vi "GetCorrdinateSysForImageArray.vi"(0 "Result data in":T2={"Measurement Names Array"=[], "Pass-Fail Array"=[], "Measurement Values Array "=[], "Roi for overlay (Arrows) Array"=[], "Algo Type Array"=[], "Image Array"=[], "Clamp operations"=enum."Average Clamp", "  Search Direction "=[], "Images_Array_in"=[], "ResultPF"=FALSE, "Total Cluster Values"={"Total Fail"=0, "Total Pass"=0, "Total Count"=0}, "Reel Counter Cluster"={"Reel Fail"=0, "Reel Pass"=0, "Reel Count"=0}, "Tolerance  Array"=[], "Array of Cam Spec Control Bool"=[], "Control Pass Fail Array"=[], "Specification Pass Fail Array"=[], "Overlay Arrow Lines"=[], "Camera ID"=[], "Trigger count"=0, "Specification fail?"=FALSE}, 2 "ImageStreams":T4, 6 "error in":errorcluster) -> (21 "Co ordinate Other":T1, 22 "Co-Ordinate System":T5(array[cluster]), 25 "Result data out":T2={"Measurement Names Array"=[], "Pass-Fail Array"=[], "Measurement Values Array "=[], "Roi for overlay (Arrows) Array"=[], "Algo Type Array"=[], "Image Array"=[], "Clamp operations"=enum."Average Clamp", "  Search Direction "=[], "Images_Array_in"=[], "ResultPF"=FALSE, "Total Cluster Values"={"Total Fail"=0, "Total Pass"=0, "Total Count"=0}, "Reel Counter Cluster"={"Reel Fail"=0, "Reel Pass"=0, "Reel Count"=0}, "Tolerance  Array"=[], "Array of Cam Spec Control Bool"=[], "Control Pass Fail Array"=[], "Specification Pass Fail Array"=[], "Overlay Arrow Lines"=[], "Camera ID"=[], "Trigger count"=0, "Specification fail?"=FALSE}, 26 "error out":errorcluster)   [LabVIEW 2019, in "Algorithm.lvclass"]
uses:
  FrameworkOverrides/Algorithm.lvclass
  <vilib>/vision/Measure.llb/Edge Polarity.ctl
  <vilib>/vision/Measure.llb/Edge Options.ctl
  Controls/Result Cluster.ctl
  Controls/ImageStreams Type Def.ctl
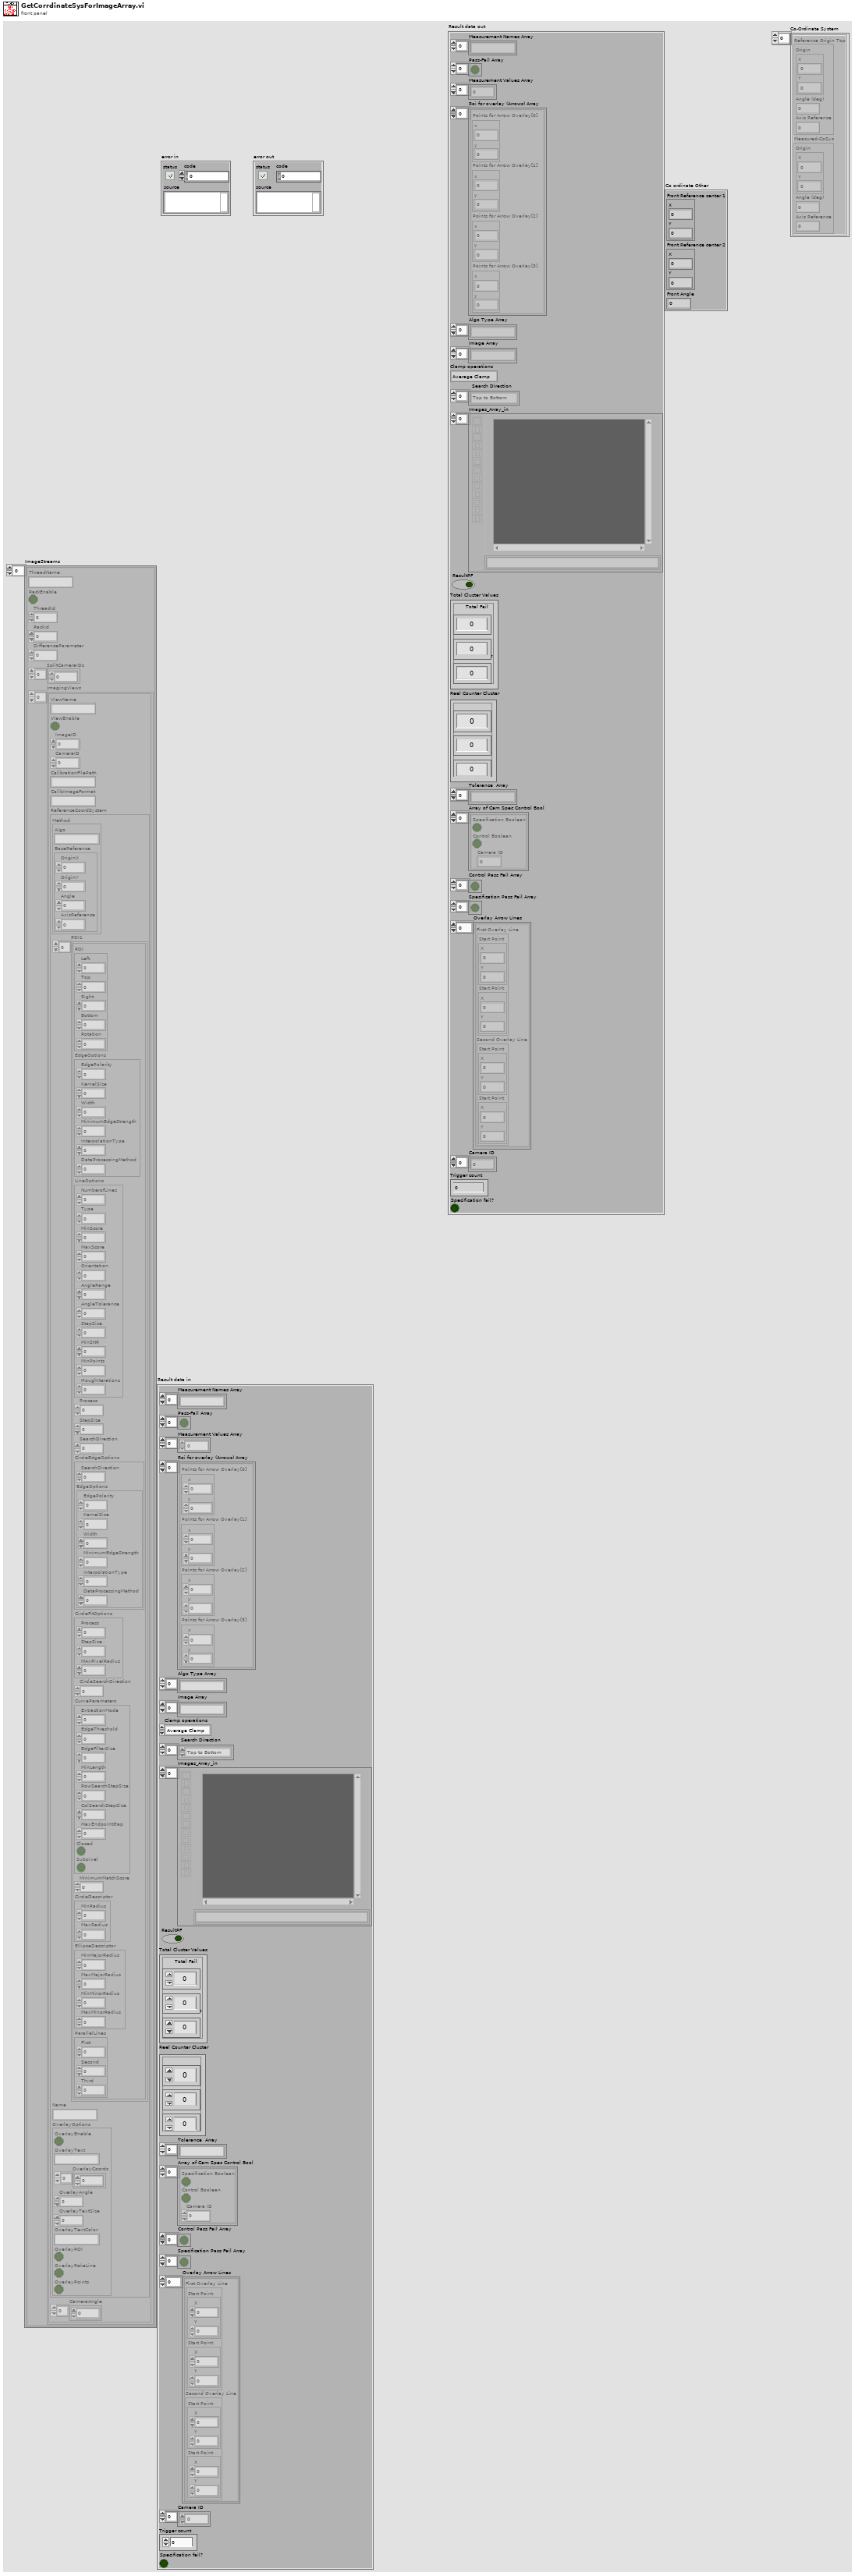
[diagram p1: front panel]
types:
  T1 = cluster{"Front Reference center 1":cluster{"X":sgl, "Y":sgl}, "Front Reference center 2":cluster{"X":sgl, "Y":sgl}, "Front Angle":dbl}
  T2 = typedef "Algorithm.lvclass/Result Cluster.ctl" = cluster{"Measurement Names Array":string[], "Pass-Fail Array":bool[], "Measurement Values Array ":dbl[], "Roi for overlay (Arrows) Array":cluster{"Points for Arrow Overlay[0]":cluster{"x":dbl, "y":dbl}, "Points for Arrow Overlay[1]":cluster{"x":dbl, "y":dbl}, "Points for Arrow Overlay[2]":cluster{"x":dbl, "y":dbl}, "Points for Arrow Overlay[3]":cluster{"x":dbl, "y":dbl}}[], "Algo Type Array":string[], "Image Array":string[], "Clamp operations":enum16{"Min Clamp", "Max Clamp", "Average Clamp"}, "  Search Direction ":enum16{"Left to Right", "Right to Left", "Top to Bottom", "Bottom to Top"}[], "Images_Array_in":T3[], "ResultPF":bool, "Total Cluster Values":cluster{"Total Fail":u64, "Total Pass":u64, "Total Count":u64}, "Reel Counter Cluster":cluster{"Reel Fail":u64, "Reel Pass":u64, "Reel Count":u64}, "Tolerance  Array":string[], "Array of Cam Spec Control Bool":cluster{"Specification Boolean":bool, "Control Boolean":bool, "Camera ID":i8}[], "Control Pass Fail Array":bool[], "Specification Pass Fail Array":bool[], "Overlay Arrow Lines":cluster{"First Overlay Line ":cluster{"Start Point":cluster{"X":sgl, "Y":sgl}, "Start Point":cluster{"X":sgl, "Y":sgl}}, "Second Overlay Line ":cluster{"Start Point":cluster{"X":sgl, "Y":sgl}, "Start Point":cluster{"X":sgl, "Y":sgl}}}[], "Camera ID":i8[], "Trigger count":i32, "Specification fail?":bool}
  T3 = typedef "IMAQ Image.ctl" = refnum<image>
  T4 = typedef "Algorithm.lvclass/ImageStreams Type Def.ctl" = cluster{"ThreadName":string, "RackEnable":bool, "ThreadId":i32, "RackId":i32, "DifferenceParameter":i32, "SplitCameraIDs":i32[], "ImagingViews":cluster{"ViewName":string, "ViewEnable":bool, "ImageID":i32, "CameraID":i32, "CalibrationFilePath":string, "CalibImageFormat":string, "ReferenceCoordSystem":cluster{"Method":cluster{"Algo":string, "BaseReference":cluster{"OriginX":i32, "OriginY":i32, "Angle":dbl, "AxisReference":i32}}, "ROI1":cluster{"ROI":cluster{"Left":i32, "Top":i32, "Right":i32, "Bottom":i32, "Rotation":dbl}, "EdgeOptions":cluster{"EdgePolarity":i32, "KernelSize":i32, "Width":i32, "MinimumEdgeStrength":i32, "InterpolationType":i32, "DataProcessingMethod":i32}, "LineOptions":cluster{"NumberofLines":i32, "Type":i32, "MinScore":i32, "MaxScore":i32, "Orientation":i32, "AngleRange":i32, "AngleTolerance":i32, "StepSize":i32, "MinSNR":i32, "MinPoints":i32, "HoughIterations":i32}, "Process":i32, "StepSize":i32, "SearchDirection":i32, "CircleEdgeOptions":cluster{"SearchDirection":i32, "EdgeOptions":cluster{"EdgePolarity":i32, "KernelSize":i32, "Width":i32, "MinimumEdgeStrength":i32, "InterpolationType":i32, "DataProcessingMethod":i32}}, "CircleFitOptions":cluster{"Process":i32, "StepSize":i32, "MAxPixelRadius":i32}, "CircleSearchDirection":i32, "CurveParameters":cluster{"ExtractionMode":i32, "EdgeThreshold":i32, "EdgeFilterSize":i32, "MinLength":i32, "RowSearchStepSize":i32, "ColSearchStepSize":i32, "MaxEndpointGap":i32, "Closed":bool, "Subpixel":bool}, "MinimumMatchScore":i32, "CircleDescriptor":cluster{"MinRadius":i32, "MaxRadius":i32}, "EllipseDescriptor":cluster{"MinMajorRadius":i32, "MaxMajorRadius":i32, "MinMinorRadius":i32, "MaxMinorRadius":i32}, "ParallelLines":cluster{"First":i32, "Second":i32, "Third":i32}}[], "Name":string, "OverlayOptions":cluster{"OverlayEnable":bool, "OverlayText":string, "OverlayCoords":i32[], "OverlayAngle":i32, "OverlayTextSize":i32, "OverlayTextColor":string, "OverlayROI":bool, "OverlayRakeLine":bool, "OverlayPoints":bool}}, "CameraAngle":dbl[]}[]}[]
  T5 = cluster{"Reference Origin Top":cluster{"Origin":cluster{"X":sgl, "Y":sgl}, "Angle (deg)":sgl, "Axis Reference":u32}, "Measured-CoSys":cluster{"Origin":cluster{"X":sgl, "Y":sgl}, "Angle (deg)":sgl, "Axis Reference":u32}}[]
  T6 = cluster{"ThreadName":string, "RackEnable":bool, "ThreadId":i32, "RackId":i32, "DifferenceParameter":i32, "SplitCameraIDs":i32[], "ImagingViews":cluster{"ViewName":string, "ViewEnable":bool, "ImageID":i32, "CameraID":i32, "CalibrationFilePath":string, "CalibImageFormat":string, "ReferenceCoordSystem":cluster{"Method":cluster{"Algo":string, "BaseReference":cluster{"OriginX":i32, "OriginY":i32, "Angle":dbl, "AxisReference":i32}}, "ROI1":cluster{"ROI":cluster{"Left":i32, "Top":i32, "Right":i32, "Bottom":i32, "Rotation":dbl}, "EdgeOptions":cluster{"EdgePolarity":i32, "KernelSize":i32, "Width":i32, "MinimumEdgeStrength":i32, "InterpolationType":i32, "DataProcessingMethod":i32}, "LineOptions":cluster{"NumberofLines":i32, "Type":i32, "MinScore":i32, "MaxScore":i32, "Orientation":i32, "AngleRange":i32, "AngleTolerance":i32, "StepSize":i32, "MinSNR":i32, "MinPoints":i32, "HoughIterations":i32}, "Process":i32, "StepSize":i32, "SearchDirection":i32, "CircleEdgeOptions":cluster{"SearchDirection":i32, "EdgeOptions":cluster{"EdgePolarity":i32, "KernelSize":i32, "Width":i32, "MinimumEdgeStrength":i32, "InterpolationType":i32, "DataProcessingMethod":i32}}, "CircleFitOptions":cluster{"Process":i32, "StepSize":i32, "MAxPixelRadius":i32}, "CircleSearchDirection":i32, "CurveParameters":cluster{"ExtractionMode":i32, "EdgeThreshold":i32, "EdgeFilterSize":i32, "MinLength":i32, "RowSearchStepSize":i32, "ColSearchStepSize":i32, "MaxEndpointGap":i32, "Closed":bool, "Subpixel":bool}, "MinimumMatchScore":i32, "CircleDescriptor":cluster{"MinRadius":i32, "MaxRadius":i32}, "EllipseDescriptor":cluster{"MinMajorRadius":i32, "MaxMajorRadius":i32, "MinMinorRadius":i32, "MaxMinorRadius":i32}, "ParallelLines":cluster{"First":i32, "Second":i32, "Third":i32}}[], "Name":string, "OverlayOptions":cluster{"OverlayEnable":bool, "OverlayText":string, "OverlayCoords":i32[], "OverlayAngle":i32, "OverlayTextSize":i32, "OverlayTextColor":string, "OverlayROI":bool, "OverlayRakeLine":bool, "OverlayPoints":bool}}, "CameraAngle":dbl[]}[]}
  T7 = cluster{"ViewName":string, "ViewEnable":bool, "ImageID":i32, "CameraID":i32, "CalibrationFilePath":string, "CalibImageFormat":string, "ReferenceCoordSystem":cluster{"Method":cluster{"Algo":string, "BaseReference":cluster{"OriginX":i32, "OriginY":i32, "Angle":dbl, "AxisReference":i32}}, "ROI1":cluster{"ROI":cluster{"Left":i32, "Top":i32, "Right":i32, "Bottom":i32, "Rotation":dbl}, "EdgeOptions":cluster{"EdgePolarity":i32, "KernelSize":i32, "Width":i32, "MinimumEdgeStrength":i32, "InterpolationType":i32, "DataProcessingMethod":i32}, "LineOptions":cluster{"NumberofLines":i32, "Type":i32, "MinScore":i32, "MaxScore":i32, "Orientation":i32, "AngleRange":i32, "AngleTolerance":i32, "StepSize":i32, "MinSNR":i32, "MinPoints":i32, "HoughIterations":i32}, "Process":i32, "StepSize":i32, "SearchDirection":i32, "CircleEdgeOptions":cluster{"SearchDirection":i32, "EdgeOptions":cluster{"EdgePolarity":i32, "KernelSize":i32, "Width":i32, "MinimumEdgeStrength":i32, "InterpolationType":i32, "DataProcessingMethod":i32}}, "CircleFitOptions":cluster{"Process":i32, "StepSize":i32, "MAxPixelRadius":i32}, "CircleSearchDirection":i32, "CurveParameters":cluster{"ExtractionMode":i32, "EdgeThreshold":i32, "EdgeFilterSize":i32, "MinLength":i32, "RowSearchStepSize":i32, "ColSearchStepSize":i32, "MaxEndpointGap":i32, "Closed":bool, "Subpixel":bool}, "MinimumMatchScore":i32, "CircleDescriptor":cluster{"MinRadius":i32, "MaxRadius":i32}, "EllipseDescriptor":cluster{"MinMajorRadius":i32, "MaxMajorRadius":i32, "MinMinorRadius":i32, "MaxMinorRadius":i32}, "ParallelLines":cluster{"First":i32, "Second":i32, "Third":i32}}[], "Name":string, "OverlayOptions":cluster{"OverlayEnable":bool, "OverlayText":string, "OverlayCoords":i32[], "OverlayAngle":i32, "OverlayTextSize":i32, "OverlayTextColor":string, "OverlayROI":bool, "OverlayRakeLine":bool, "OverlayPoints":bool}}, "CameraAngle":dbl[]}[]
  T8 = cluster{"Origin":cluster{"X":sgl, "Y":sgl}, "Angle (deg)":sgl, "Axis Reference":u32}
  T9 = cluster{"Base Reference":cluster{"Origin":cluster{"X":sgl, "Y":sgl}, "Angle (deg)":sgl, "Axis Reference":u32}, "New Reference":cluster{"Origin":cluster{"X":sgl, "Y":sgl}, "Angle (deg)":sgl, "Axis Reference":u32}}
  T10 = typedef "Edge Options.ctl" = cluster{"Edge Polarity":T11, "Kernel Size":u32, "Width":u32, "Minimum Edge Strength":sgl, "Interpolation Type":enum32{"Zero Order", "Bilinear", "Quadratic", "Cubic", "Bilinear Fixed"}, "Data Processing Method":enum32{"Average", "Median"}}
  T11 = typedef "Edge Polarity.ctl" = u32
  T12 = cluster{"Search Direction":u32, "Edge Options":T10, "Show Search Area":bool, "Show Search Lines":bool, "Show Edges Found":bool, "Show Result":bool, "Search Area Color":u32, "Search Lines Color":u32, "Edge Locations Color":u32, "Result Color":u32, "Overlay Group Name":string}
  T13 = cluster{"Area Lower Value":dbl, "Area Upper Value":dbl}
  T14 = cluster{"Method":cluster{"Algo":string, "BaseReference":cluster{"OriginX":i32, "OriginY":i32, "Angle":dbl, "AxisReference":i32}}, "ROI1":cluster{"ROI":cluster{"Left":i32, "Top":i32, "Right":i32, "Bottom":i32, "Rotation":dbl}, "EdgeOptions":cluster{"EdgePolarity":i32, "KernelSize":i32, "Width":i32, "MinimumEdgeStrength":i32, "InterpolationType":i32, "DataProcessingMethod":i32}, "LineOptions":cluster{"NumberofLines":i32, "Type":i32, "MinScore":i32, "MaxScore":i32, "Orientation":i32, "AngleRange":i32, "AngleTolerance":i32, "StepSize":i32, "MinSNR":i32, "MinPoints":i32, "HoughIterations":i32}, "Process":i32, "StepSize":i32, "SearchDirection":i32, "CircleEdgeOptions":cluster{"SearchDirection":i32, "EdgeOptions":cluster{"EdgePolarity":i32, "KernelSize":i32, "Width":i32, "MinimumEdgeStrength":i32, "InterpolationType":i32, "DataProcessingMethod":i32}}, "CircleFitOptions":cluster{"Process":i32, "StepSize":i32, "MAxPixelRadius":i32}, "CircleSearchDirection":i32, "CurveParameters":cluster{"ExtractionMode":i32, "EdgeThreshold":i32, "EdgeFilterSize":i32, "MinLength":i32, "RowSearchStepSize":i32, "ColSearchStepSize":i32, "MaxEndpointGap":i32, "Closed":bool, "Subpixel":bool}, "MinimumMatchScore":i32, "CircleDescriptor":cluster{"MinRadius":i32, "MaxRadius":i32}, "EllipseDescriptor":cluster{"MinMajorRadius":i32, "MaxMajorRadius":i32, "MinMinorRadius":i32, "MaxMinorRadius":i32}, "ParallelLines":cluster{"First":i32, "Second":i32, "Third":i32}}[], "Name":string, "OverlayOptions":cluster{"OverlayEnable":bool, "OverlayText":string, "OverlayCoords":i32[], "OverlayAngle":i32, "OverlayTextSize":i32, "OverlayTextColor":string, "OverlayROI":bool, "OverlayRakeLine":bool, "OverlayPoints":bool}}
  T15 = cluster{"Algo":string, "BaseReference":cluster{"OriginX":i32, "OriginY":i32, "Angle":dbl, "AxisReference":i32}}
  T16 = cluster{"ROI":cluster{"Left":i32, "Top":i32, "Right":i32, "Bottom":i32, "Rotation":dbl}, "EdgeOptions":cluster{"EdgePolarity":i32, "KernelSize":i32, "Width":i32, "MinimumEdgeStrength":i32, "InterpolationType":i32, "DataProcessingMethod":i32}, "LineOptions":cluster{"NumberofLines":i32, "Type":i32, "MinScore":i32, "MaxScore":i32, "Orientation":i32, "AngleRange":i32, "AngleTolerance":i32, "StepSize":i32, "MinSNR":i32, "MinPoints":i32, "HoughIterations":i32}, "Process":i32, "StepSize":i32, "SearchDirection":i32, "CircleEdgeOptions":cluster{"SearchDirection":i32, "EdgeOptions":cluster{"EdgePolarity":i32, "KernelSize":i32, "Width":i32, "MinimumEdgeStrength":i32, "InterpolationType":i32, "DataProcessingMethod":i32}}, "CircleFitOptions":cluster{"Process":i32, "StepSize":i32, "MAxPixelRadius":i32}, "CircleSearchDirection":i32, "CurveParameters":cluster{"ExtractionMode":i32, "EdgeThreshold":i32, "EdgeFilterSize":i32, "MinLength":i32, "RowSearchStepSize":i32, "ColSearchStepSize":i32, "MaxEndpointGap":i32, "Closed":bool, "Subpixel":bool}, "MinimumMatchScore":i32, "CircleDescriptor":cluster{"MinRadius":i32, "MaxRadius":i32}, "EllipseDescriptor":cluster{"MinMajorRadius":i32, "MaxMajorRadius":i32, "MinMinorRadius":i32, "MaxMinorRadius":i32}, "ParallelLines":cluster{"First":i32, "Second":i32, "Third":i32}}[]
  T17 = cluster{"OverlayEnable":bool, "OverlayText":string, "OverlayCoords":i32[], "OverlayAngle":i32, "OverlayTextSize":i32, "OverlayTextColor":string, "OverlayROI":bool, "OverlayRakeLine":bool, "OverlayPoints":bool}
  T18 = cluster{"OriginX":i32, "OriginY":i32, "Angle":dbl, "AxisReference":i32}
  T19 = cluster{"ROI":cluster{"Left":i32, "Top":i32, "Right":i32, "Bottom":i32, "Rotation":dbl}, "EdgeOptions":cluster{"EdgePolarity":i32, "KernelSize":i32, "Width":i32, "MinimumEdgeStrength":i32, "InterpolationType":i32, "DataProcessingMethod":i32}, "LineOptions":cluster{"NumberofLines":i32, "Type":i32, "MinScore":i32, "MaxScore":i32, "Orientation":i32, "AngleRange":i32, "AngleTolerance":i32, "StepSize":i32, "MinSNR":i32, "MinPoints":i32, "HoughIterations":i32}, "Process":i32, "StepSize":i32, "SearchDirection":i32, "CircleEdgeOptions":cluster{"SearchDirection":i32, "EdgeOptions":cluster{"EdgePolarity":i32, "KernelSize":i32, "Width":i32, "MinimumEdgeStrength":i32, "InterpolationType":i32, "DataProcessingMethod":i32}}, "CircleFitOptions":cluster{"Process":i32, "StepSize":i32, "MAxPixelRadius":i32}, "CircleSearchDirection":i32, "CurveParameters":cluster{"ExtractionMode":i32, "EdgeThreshold":i32, "EdgeFilterSize":i32, "MinLength":i32, "RowSearchStepSize":i32, "ColSearchStepSize":i32, "MaxEndpointGap":i32, "Closed":bool, "Subpixel":bool}, "MinimumMatchScore":i32, "CircleDescriptor":cluster{"MinRadius":i32, "MaxRadius":i32}, "EllipseDescriptor":cluster{"MinMajorRadius":i32, "MaxMajorRadius":i32, "MinMinorRadius":i32, "MaxMinorRadius":i32}, "ParallelLines":cluster{"First":i32, "Second":i32, "Third":i32}}
  T20 = cluster{"Left":i32, "Top":i32, "Right":i32, "Bottom":i32, "Rotation":dbl}
  T21 = typedef "ROI Descriptor" = cluster{"Global Rectangle":i32[], "Contours":cluster{"ID":enum32{"External", "Internal"}, "Type":u32, "Coordinates":i32[]}[]}
  T22 = cluster{"NumberofLines":i32, "Type":i32, "MinScore":i32, "MaxScore":i32, "Orientation":i32, "AngleRange":i32, "AngleTolerance":i32, "StepSize":i32, "MinSNR":i32, "MinPoints":i32, "HoughIterations":i32}
  T23 = cluster{"EdgePolarity":i32, "KernelSize":i32, "Width":i32, "MinimumEdgeStrength":i32, "InterpolationType":i32, "DataProcessingMethod":i32}
  T24 = cluster{"MinMajorRadius":i32, "MaxMajorRadius":i32, "MinMinorRadius":i32, "MaxMinorRadius":i32}
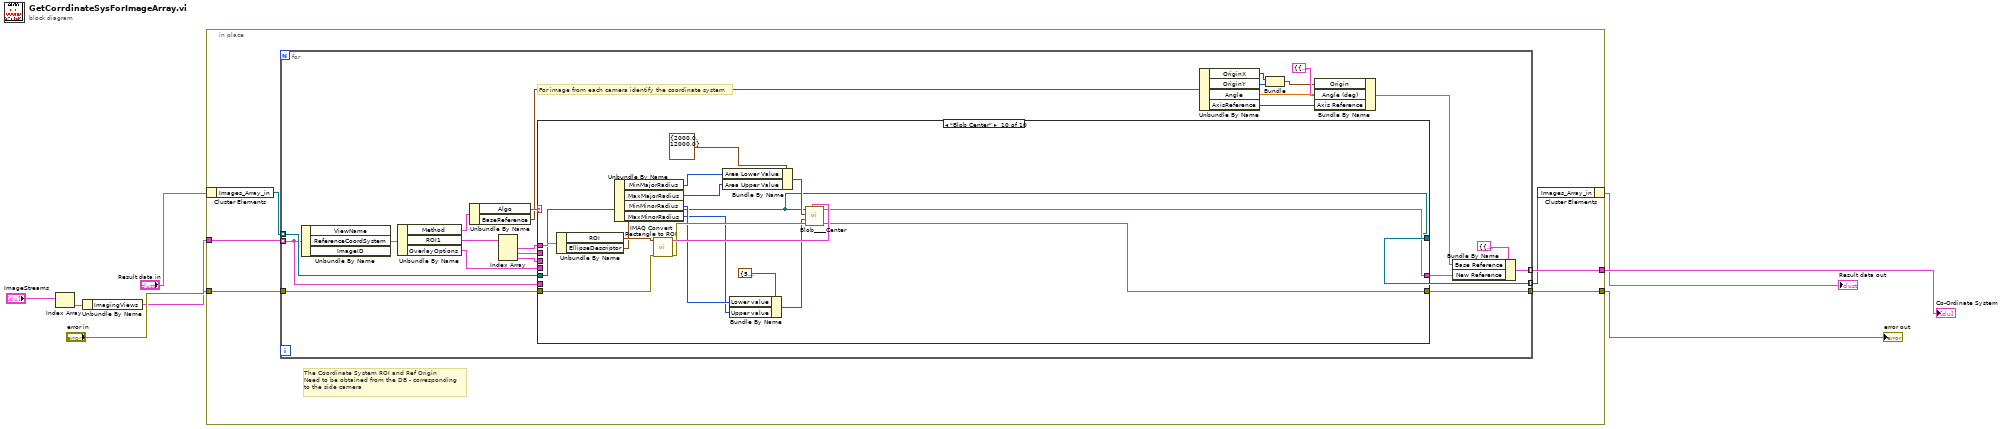
[diagram p0: block diagram]
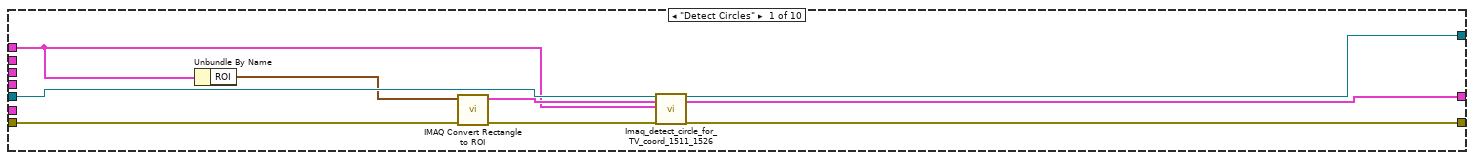
[diagram p2: hidden frame]
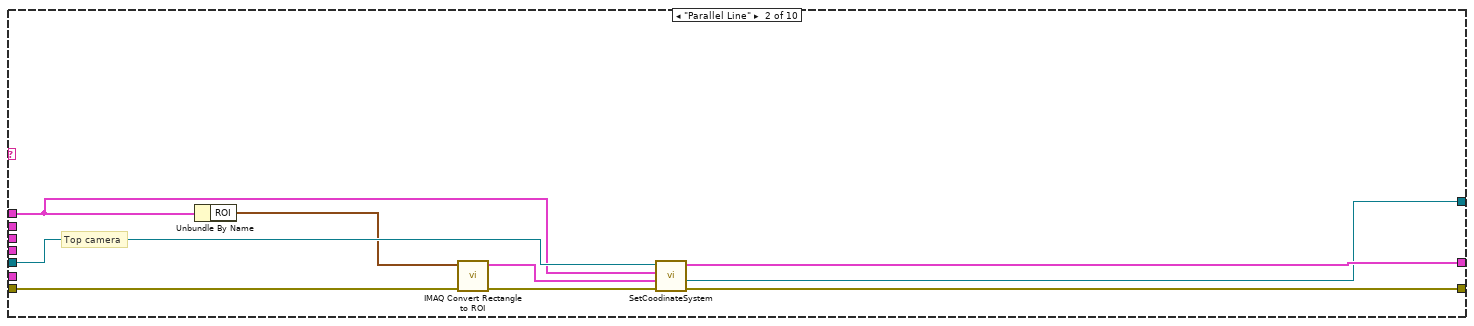
[diagram p3: hidden frame]
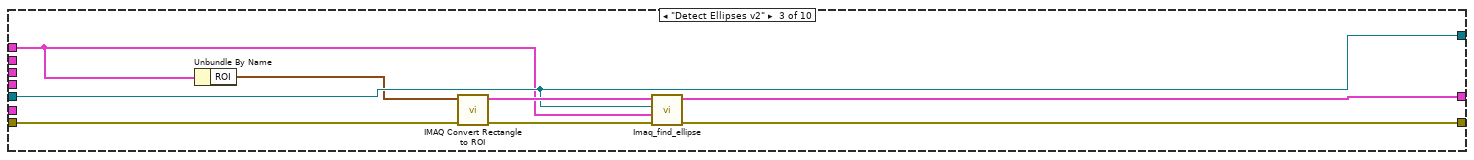
[diagram p4: hidden frame]
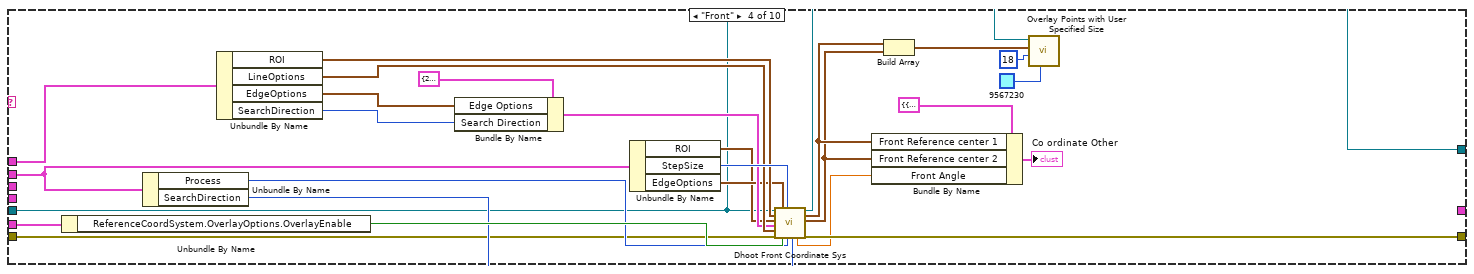
[diagram p5: hidden frame]
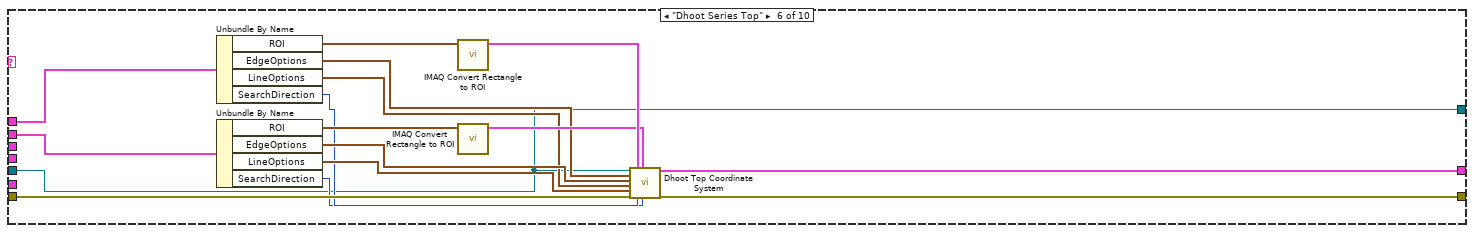
[diagram p7: hidden frame]
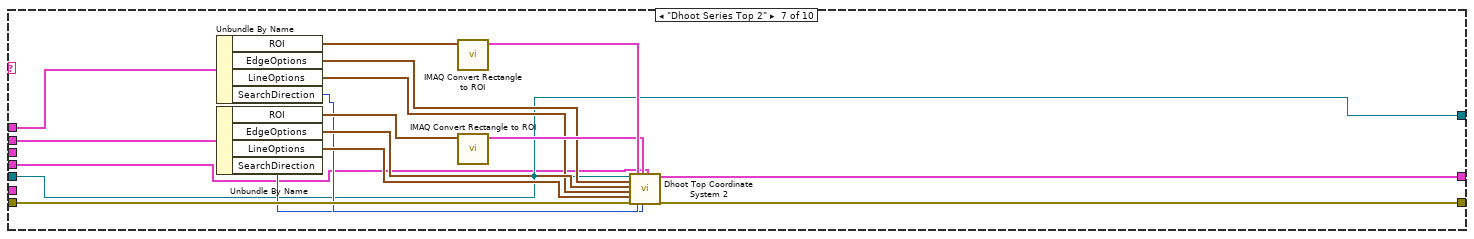
[diagram p8: hidden frame]
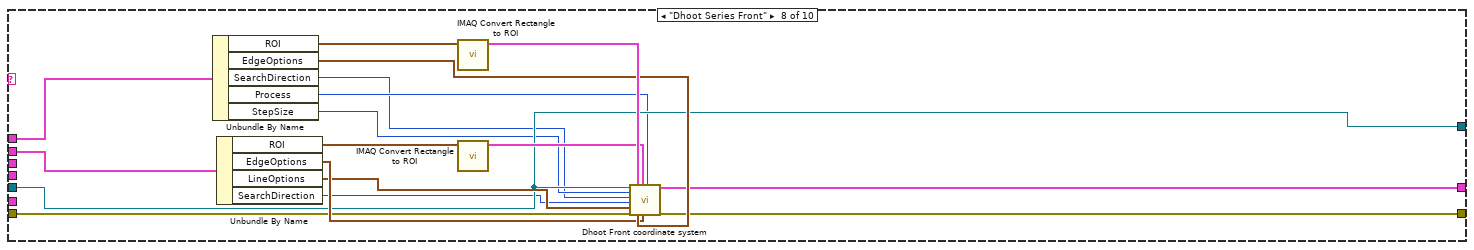
[diagram p9: hidden frame]
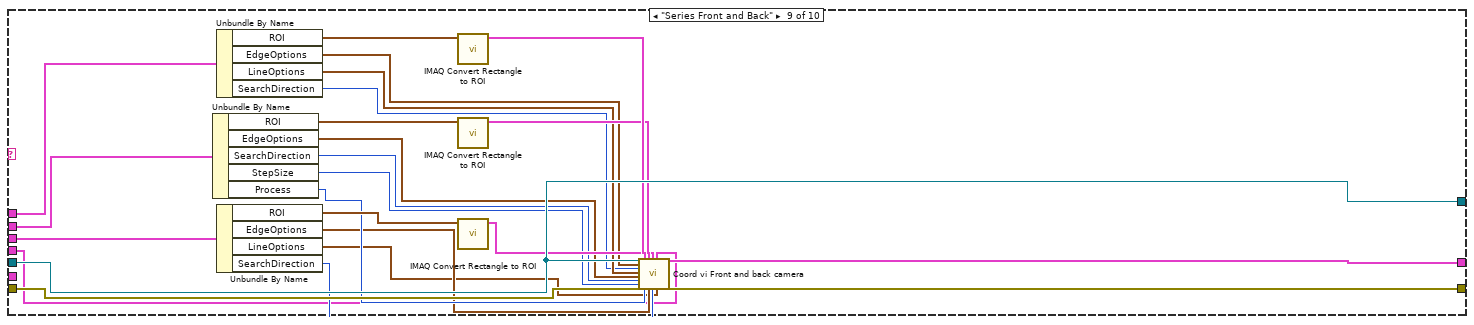
[diagram p10: hidden frame]
diagram:
  n1 = Index Array(array="ImageStreams") -> (element=w5:T6)  [unwired: 1 in]
  n2 = Unbundle By Name(w5) -> ("ImagingViews"=w4:T7)
  n3 = in-place {
    in-place-border: "error in" -> [w14]
    in-place-border: [w13] -> w7
    in-place-border: [w12] -> w6
    in-place-border: w4 -> [w11]
    # "The Coordinate System ROI and Ref Origin\nNeed to be obtained from the DB - corresponding\nto the side camera"
    n4 = in-place-cluster #1("Result data in") -> ("Images_Array_in"=w10:T3[])
    n5 = for {
      tunnel: w14 -> [w38]
      tunnel: w10 -> [w37] mode=indexing
      tunnel: [w36] -> w13
      tunnel: [w35] -> w9 mode=indexing
      tunnel: [w33] -> w12 mode=indexing
      tunnel: w11 -> [w19] mode=indexing
      # "For image from each camera identify the coordinate system"
      n6 = Unbundle By Name(w19) -> ("ReferenceCoordSystem"=w32:T14)  [unwired: 2 out]
      n7 = Unbundle By Name(w32) -> ("Method"=w31:T15, "ROI1"=w21:T16, "OverlayOptions"=w15:T17)
      n8 = Unbundle By Name(w31) -> ("Algo"=w30:string, "BaseReference"=w29:T18)
      n9 = Index Array(array=w21) -> (element #1=w22:T19, element #2=w20:T19, element #3=w17:T19)  [unwired: 3 in]
      n10 = case shown="\"Blob Center\"" w30 {
        tunnel: w38 -> [w45 w54 w63 w77 w93 w109 w126 w134 w164 w181]
        tunnel: [w42 w51 w62 w76 w93 w108 w125 w133 w165 w170] -> w36
        tunnel: [w43 w50 w60 w75 w92 w94 w111 w131 w166 w168] -> w35
        tunnel: w37 -> [w44 w53 w60 w73 w92 w94 w111 w131 w166 w168]
        tunnel: w20 -> [_ _ _ w79 _ w106 w123 w140 w162 _]
        tunnel: w22 -> [w40 w49 w59 w78 _ w107 w124 w143 w163 w184]
        tunnel: [w41 w52 w57 _ _ w95 w112 w132 w167 w169] -> w18
        tunnel: w19 -> [_ _ _ w74 _ _ _ _ _ _]
        tunnel: w17 -> [_ _ _ _ _ _ _ _ w161 _]
        tunnel: w15 -> [_ _ _ _ _ _ w110 _ w144 _]
        frame "Detect Circles" {
          n11 = Unbundle By Name(w40) -> ("ROI"=w39:T20)
          n12 = call "IMAQ Convert Rectangle to ROI"("error in (no error)"=w45, "Rectangle"=w39) -> ("error out"=w46:errorcluster, "ROI Descriptor"=w47:T21)  [unwired: 7 in]
          n13 = call "Imaq_detect_circle_for_TV_coord_1511_1526.vi"("Image"=w44, "ROI"=w47, "ROI1"=w40, "error in (no error)"=w46) -> ("Image Out"=w43:T3, "New Reference"=w41:T8, "error out"=w42:errorcluster)  [unwired: 13 in]
        }
        frame "Parallel Line" {
          # "Top camera"
          n14 = Unbundle By Name(w49) -> ("ROI"=w48:T20)
          n15 = call "IMAQ Convert Rectangle to ROI"("error in (no error)"=w54, "Rectangle"=w48) -> ("error out"=w55:errorcluster, "ROI Descriptor"=w56:T21)  [unwired: 7 in]
          n16 = call "SetCoodinateSystem.vi"("error in"=w55, "ROI Descriptor"=w56, "ROI1"=w49, "Refnum in"=w53) -> ("error out"=w51:errorcluster, "Image Out"=w50:T3, "Coordinate System"=w52:T8)  [unwired: 5 in]
        }
        frame "Detect Ellipses v2" {
          n17 = Unbundle By Name(w59) -> ("ROI"=w58:T20)
          n18 = call "IMAQ Convert Rectangle to ROI"("error in (no error)"=w63, "Rectangle"=w58) -> ("error out"=w64:errorcluster, "ROI Descriptor"=w61:T21)  [unwired: 7 in]
          n19 = call "Imaq_find_ellipse.vi"("error in (no error)"=w64, "ROI1"=w59, "Image In"=w60, "ROI Descriptor"=w61) -> ("error out"=w62:errorcluster, "New Reference"=w57:T8)  [unwired: 6 in]
        }
        frame "Front" {
          n20 = Unbundle By Name(w74) -> ("ReferenceCoordSystem.OverlayOptions.OverlayEnable"=w91:bool)
          n21 = Unbundle By Name(w79) -> ("Process"=w89:i32, "SearchDirection"=w90:i32)
          n22 = Unbundle By Name(w78) -> ("ROI"=w87:T20, "LineOptions"=w86:T22, "EdgeOptions"=w83:T23, "SearchDirection"=w84:i32)
          n23 = Bundle By Name(cluster=T12 {"Search Direction"=2, "Edge Options"={"Edge Polarity"=0, "Kernel Size"=7, "Width"=7, "Minimum Edge Strength"=40.0, "Interpolation Type"=enum."Zero Order", "Data Processing Method"=enum."Average"}, "Show Search Area"=FALSE, "Show Search Lines"=FALSE, "Show Edges Found"=FALSE, "Show Result"=TRUE, "Search Area Color"=65280, "Search Lines Color"=255, "Edge Locations Color"=16776960, "Result Color"=16711680, "Overlay Group Name"=""} ("Options"), "Edge Options"=w83, "Search Direction"=w84) -> (w85:T12)
          n24 = Unbundle By Name(w79) -> ("ROI"=w80:T20, "StepSize"=w88:i32, "EdgeOptions"=w82:T23)
          n25 = call "Dhoot Front Coordinate Sys.vi"("Image Out"=w73, "First Reference ROI"=w87, "Second Reference ROI"=w80, "Options"=w85, "Line Fit Options"=w86, "error in (no error)"=w77, "Edge Options"=w82, "ROI Enable True/False"=w91, "Step Size"=w88, "Process"=w89, "Scan Direction"=w90) -> ("Angle (Pixel)"=w67:dbl, "Image Out"=w75:T3, "First Reference Centre"=w69:cluster{"Centre X":dbl, "Centre Y":dbl}, "Second Reference Centre"=w68:cluster{"Centre X":dbl, "Centre Y":dbl}, "error IO"=w76:errorcluster)  [unwired: 4 in]
          n26 = Bundle By Name(cluster=T1 {"Front Reference center 1"={"X"=0.0, "Y"=0.0}, "Front Reference center 2"={"X"=0.0, "Y"=0.0}, "Front Angle"=0.0} ("Coordinate Other Cluster"), "Front Reference center 1"=w69, "Front Reference center 2"=w68, "Front Angle"=w67) -> (→"Co ordinate Other":T1)
          n27 = Build Array(w69, w68) -> (w72:cluster{"Centre X":dbl, "Centre Y":dbl}[])
          n28 = call "Overlay Points with User Specified Size.vi"("Color"=u32 9567230, "Point Diameter (5)"=u32 18, "Points"=w72, "Image In"=w73) -> ()  [unwired: 6 in, 2 out]
        }
        frame "", Default {
        }
        frame "Dhoot Series Top" {
          n29 = Unbundle By Name(w107) -> ("ROI"=w105:T20, "EdgeOptions"=w101:T23, "LineOptions"=w99:T22, "SearchDirection"=w97:i32)
          n30 = Unbundle By Name(w106) -> ("ROI"=w104:T20, "EdgeOptions"=w100:T23, "LineOptions"=w98:T22, "SearchDirection"=w96:i32)
          n31 = call "IMAQ Convert Rectangle to ROI"("Rectangle"=w105) -> ("ROI Descriptor"=w103:T21)  [unwired: 8 in, 1 out]
          n32 = call "IMAQ Convert Rectangle to ROI"("Rectangle"=w104) -> ("ROI Descriptor"=w102:T21)  [unwired: 8 in, 1 out]
          n33 = call "Dhoot Top Coordinate System.vi"("Image Out"=w94, "Edge Options ROI 1"=w101, "Edge Options ROI 2"=w100, "Line Options ROI 1"=w99, "Line Options ROI 2"=w98, "error in (no error)"=w109, "ROI 1"=w103, "Search Direction ROI 1"=w97, "ROI 2"=w102, "Search Direction ROI 2"=w96) -> ("Co ordinate System"=w95:T8, "error out"=w108:errorcluster)  [unwired: 8 in]
        }
        frame "Dhoot Series Top 2" {
          n34 = Unbundle By Name(w124) -> ("ROI"=w122:T20, "EdgeOptions"=w118:T23, "LineOptions"=w116:T22, "SearchDirection"=w114:i32)
          n35 = Unbundle By Name(w123) -> ("ROI"=w121:T20, "EdgeOptions"=w117:T23, "LineOptions"=w115:T22, "SearchDirection"=w113:i32)
          n36 = call "IMAQ Convert Rectangle to ROI"("Rectangle"=w122) -> ("ROI Descriptor"=w120:T21)  [unwired: 8 in, 1 out]
          n37 = call "IMAQ Convert Rectangle to ROI"("Rectangle"=w121) -> ("ROI Descriptor"=w119:T21)  [unwired: 8 in, 1 out]
          n38 = call "Dhoot Top Coordinate System 2.vi"("Image Out"=w111, "Edge Options ROI 1"=w118, "Edge Options ROI 2"=w117, "Line Options ROI 1"=w116, "Line Options ROI 2"=w115, "error in (no error)"=w126, "ROI 1"=w120, "Search Direction ROI 1"=w114, "ROI 2"=w119, "Search Direction ROI 2"=w113, "OverlayOptions"=w110) -> ("Co ordinate System"=w112:T8, "error out"=w125:errorcluster)  [unwired: 7 in]
        }
        frame "Dhoot Series Front" {
          n39 = Unbundle By Name(w143) -> ("ROI"=w142:T20, "EdgeOptions"=w137:T23, "SearchDirection"=w128:i32, "Process"=w130:i32, "StepSize"=w129:i32)
          n40 = Unbundle By Name(w140) -> ("ROI"=w139:T20, "EdgeOptions"=w136:T23, "LineOptions"=w135:T22, "SearchDirection"=w127:i32)
          n41 = call "IMAQ Convert Rectangle to ROI"("Rectangle"=w142) -> ("ROI Descriptor"=w141:T21)  [unwired: 8 in, 1 out]
          n42 = call "IMAQ Convert Rectangle to ROI"("Rectangle"=w139) -> ("ROI Descriptor"=w138:T21)  [unwired: 8 in, 1 out]
          n43 = call "Dhoot Front coordinate system.vi"("Image In"=w131, "Step Size ROI 1"=w129, "Scan Direction ROI 1"=w128, "Search Direction ROI 2"=w127, "Line Options ROI 2"=w135, "error in (no error)"=w134, "ROI 1"=w141, "Edge Options ROI 1"=w137, "ROI 2"=w138, "Edge Options ROI 2"=w136, "Process ROI 1"=w130) -> ("Co ordinate System"=w132:T8, "error out"=w133:errorcluster)  [unwired: 7 in]
        }
        frame "Series Front and Back" {
          n44 = Unbundle By Name(w162) -> ("ROI"=w159:T20, "EdgeOptions"=w146:T23, "SearchDirection"=w145:i32, "StepSize"=w150:i32, "Process"=w154:i32)
          n45 = Unbundle By Name(w163) -> ("ROI"=w160:T20, "EdgeOptions"=w149:T23, "LineOptions"=w148:T22, "SearchDirection"=w147:i32)
          n46 = Unbundle By Name(w161) -> ("ROI"=w158:T20, "EdgeOptions"=w153:T23, "LineOptions"=w151:T22, "SearchDirection"=w152:i32)
          n47 = call "IMAQ Convert Rectangle to ROI"("Rectangle"=w160) -> ("ROI Descriptor"=w157:T21)  [unwired: 8 in, 1 out]
          n48 = call "IMAQ Convert Rectangle to ROI"("Rectangle"=w159) -> ("ROI Descriptor"=w156:T21)  [unwired: 8 in, 1 out]
          n49 = call "IMAQ Convert Rectangle to ROI"("Rectangle"=w158) -> ("ROI Descriptor"=w155:T21)  [unwired: 8 in, 1 out]
          n50 = call "Coord vi Front and back camera.vi"("Image Out"=w166, "Edge Options"=w149, "Search Direction"=w147, "Line Options"=w148, "Edge Options ROI 2"=w146, "Scan Direction ROI 2"=w145, "Step Size ROI 2"=w150, "error in (no error)"=w164, "ROI 1"=w157, "Process ROI 2"=w154, "ROI 2"=w156, "Edge OptionsROI 3"=w153, "ROI 3"=w155, "Search Direction ROI 3"=w152, "OverlayOptions"=w144, "Line Options ROI 3"=w151) -> ("output cluster"=w167:T8, "error out"=w165:errorcluster)  [unwired: 10 in]
        }
        frame "Blob Center" {
          n51 = Unbundle By Name(w184) -> ("ROI"=w183:T20, "EllipseDescriptor"=w178:T24)
          n52 = Unbundle By Name(w178) -> ("MinMajorRadius"=w177:i32, "MaxMajorRadius"=w176:i32, "MinMinorRadius"=w174:i32, "MaxMinorRadius"=w173:i32)
          n53 = call "IMAQ Convert Rectangle to ROI"("error in (no error)"=w181, "Rectangle"=w183) -> ("error out"=w180:errorcluster, "ROI Descriptor"=w182:T21)  [unwired: 7 in]
          n54 = Bundle By Name(cluster=T13 {"Area Lower Value"=2000.0, "Area Upper Value"=12000.0} ("Area Limits Cluster"), "Area Lower Value"=w177, "Area Upper Value"=w176) -> (w172:T13)
          n55 = Bundle By Name(cluster=cluster{"Lower value":sgl, "Upper value":sgl} {"Lower value"=50.0, "Upper value"=255.0} ("Edge Strength Cluster"), "Lower value"=w174, "Upper value"=w173) -> (w171:cluster{"Lower value":sgl, "Upper value":sgl})
          n56 = call "Blob____Center.vi"("ROI"=w182, "error in (no error)"=w180, "Edge Strength Cluster"=w171, "Area Limits Cluster"=w172, "Image Out"=w168) -> ("error out"=w170:errorcluster, "Co Ordinate System"=w169:T8)  [unwired: 5 in]
        }
      }
      n57 = Unbundle By Name(w29) -> ("OriginX"=w27:i32, "OriginY"=w26:i32, "Angle"=w24:dbl, "AxisReference"=w23:i32)
      n58 = Bundle("OriginX"=w27, "OriginY"=w26) -> (w25:cluster{"OriginX":i32, "OriginY":i32})  [unwired: 1 in]
      n59 = Bundle By Name(cluster=T8 {"Origin"={"X"=0.0, "Y"=0.0}, "Angle (deg)"=0.0, "Axis Reference"=0} ("Reference Origin Top"), "Origin"=w25, "Angle (deg)"=w24, "Axis Reference"=w23) -> (w16:T8)
      n60 = Bundle By Name(cluster=T9 {"Base Reference"={"Origin"={"X"=0.0, "Y"=0.0}, "Angle (deg)"=0.0, "Axis Reference"=0}, "New Reference"={"Origin"={"X"=0.0, "Y"=0.0}, "Angle (deg)"=0.0, "Axis Reference"=0}} ("Co-Ordinate System"), "Base Reference"=w16, "New Reference"=w18) -> (w33:T9)
    }
    n61 = in-place-cluster #1("Images_Array_in"=w9) -> (→"Result data out":T2)
  }
  "error out" <- w7
  "Co-Ordinate System" <- w6
